vi "Ej8.vi"() -> ()   [LabVIEW 2023]
panel:
  out "Square Root":dbl
  out "error out":errorcluster
  in  "error in (no error)":errorcluster
  in  "Square Root Input":dbl
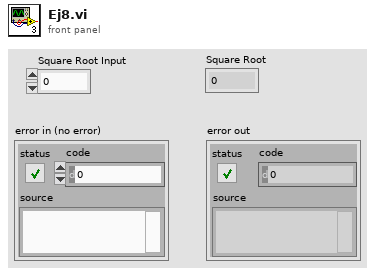
[diagram p1: front panel]
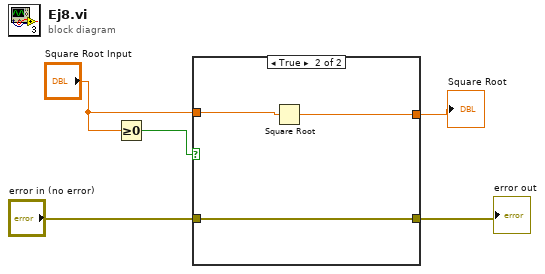
[diagram p0: block diagram]
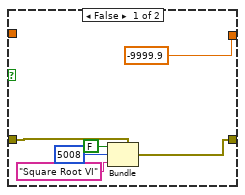
[diagram p2: hidden frame]
diagram:
  n1 = Greater Or Equal To 0?(x="Square Root Input") -> (x >= 0?=w5:bool)
  n2 = case shown="True" w5 {
    tunnel: "Square Root Input" -> [_ w14]
    tunnel: [-9999.9 w13] -> w3
    tunnel: "error in (no error)" -> [w10 w12]
    tunnel: [w9 w12] -> w1
    frame False {
      n3 = Bundle(cluster=w10, "status"=FALSE, "code"=5008, "source"="Square Root VI") -> (w9:errorcluster)
    }
    frame True {
      n4 = Square Root(x=w14) -> (sqrt(x)=w13:dbl)
    }
  }
  "error out" <- w1
  "Square Root" <- w3
